vi "graph end locations.vi"() -> ()   [LabVIEW 2009]
uses:
  arcade drive.llb/drive respect.ctl
panel:
  in  "duration (s)":dbl
  out "end points":cluster{dbl, dbl}[](graph)
  in  "speeds":cluster{"speed":dbl, "turn":dbl}[](array[cluster]) {"speed" step=0.05000000074505806 scale=-1.0..1.0; "turn" step=0.05000000074505806 scale=-1.0..1.0}
  in  "initial":T1
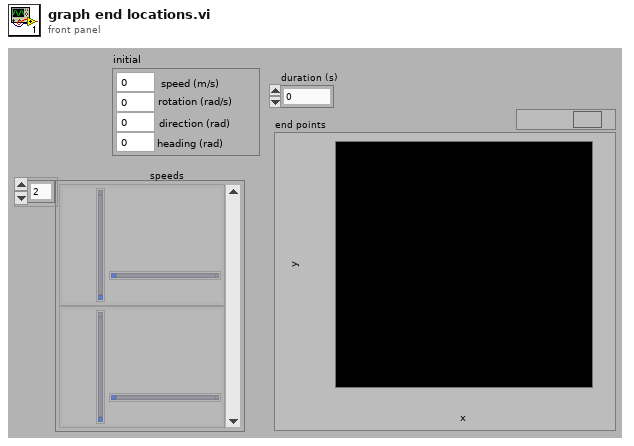
[diagram p1: front panel]
types:
  T1 = cluster{"speed (m/s)":dbl, "rotation (rad/s)":dbl, "direction (rad)":dbl, "heading (rad)":dbl}
  T2 = typedef "drive respect.ctl" = enum16{"none", "average", "turn", "speed"}
  T3 = cluster{"width (displayed)":dbl, "actual width (m)":dbl, "respect (none)":T2, "iterations/s":dbl, "maxiumum":cluster{"speed":dbl, "rotational acceleration":dbl}, "coefficient of friction":cluster{"forward":dbl, "perpendicular":dbl}, "robot start location":cluster{"x":dbl, "y":dbl}}
  T4 = cluster{"speed":dbl, "turn":dbl, "duration (s)":dbl}
  T5 = cluster{"speed":dbl, "turn":dbl, "duration (s)":dbl}[]
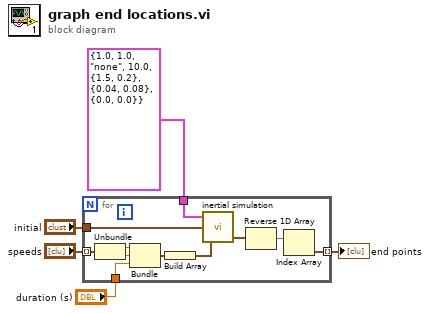
[diagram p0: block diagram]
diagram:
  n1 = for {
    tunnel: "initial" -> [w14]
    tunnel: T3 {"width (displayed)"=1.0, "actual width (m)"=1.0, "respect (none)"=enum."none", "iterations/s"=10.0, "maxiumum"={"speed"=1.5, "rotational acceleration"=0.2}, "coefficient of friction"={"forward"=0.04, "perpendicular"=0.08}, "robot start location"={"x"=0.0, "y"=0.0}} ("configuration") -> [w13]
    tunnel: "speeds" -> [w11] mode=indexing
    tunnel: [w12] -> w3 mode=indexing
    tunnel: "duration (s)" -> [w6]
    n2 = Unbundle(w11) -> ("speed"=w10:dbl, "turn"=w9:dbl)
    n3 = Bundle("speed"=w10, "turn"=w9, "duration (s)"=w6) -> (w8:T4)  [unwired: 1 in]
    n4 = Build Array(w8) -> (w7:T5)
    n5 = call "inertial simulation.vi"("speeds"=w7, "initial"=w14, "configuration"=w13) -> ("locations"=w16:cluster{dbl, dbl}[])  [unwired: 1 in, 1 out]
    n6 = Reverse 1D Array(array=w16) -> (reversed array=w15:cluster{dbl, dbl}[])
    n7 = Index Array(array=w15) -> (element=w12:cluster{dbl, dbl})  [unwired: 1 in]
  }
  "end points" <- w3
